vi "Untitled 1.vi"() -> ()   [LabVIEW 2016]
uses:
  Control 1.ctl
panel:
  out "Gauge":i32(knob) scale=0.0..100.0
  out "Numeric 2":dbl
  out "Numeric":T1
  in  "Slide":dbl(slide) scale=0.0..10.0
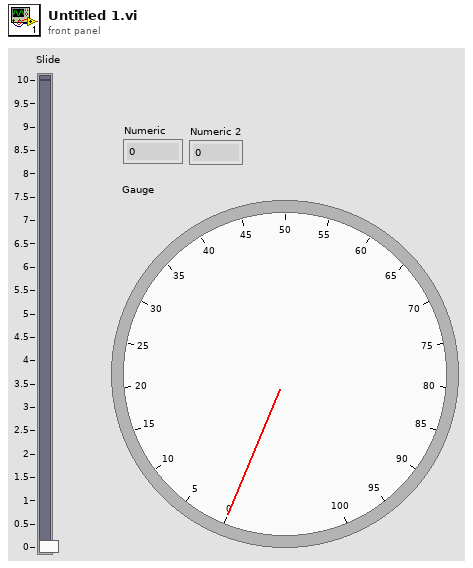
[diagram p1: front panel]
types:
  T1 = typedef "Control 1.ctl" = dbl
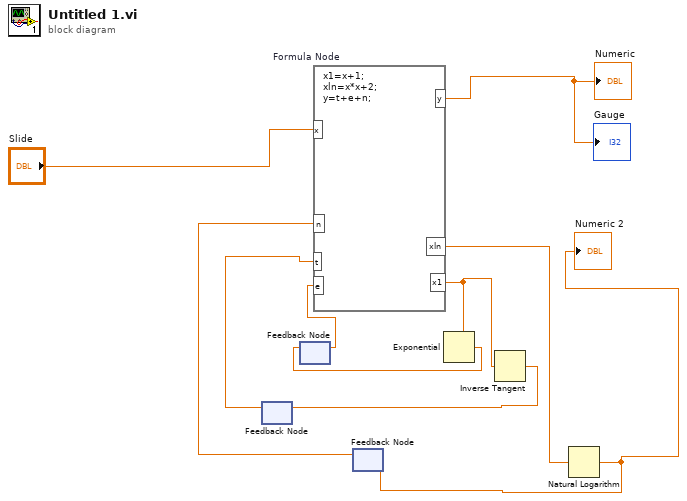
[diagram p0: block diagram]
diagram:
  n1 = feedback #1() -> (w3:dbl)  [unwired: 1 in]
  n2 = feedback #2() -> (w5:dbl)  [unwired: 1 in]
  n3 = feedback #3() -> (w2:dbl)  [unwired: 1 in]
  n4 = formula code="x1=x+1;\nxln=x*x+2;\ny=t+e+n;"("x"="Slide", "t"=w3, "e"=w5, "n"=w2) -> ("y"=→"Numeric" →"Gauge":dbl, "x1"=w7:dbl, "xln"=w8:dbl)
  n5 = Exponential(1:w7) -> (0:w6:dbl)
  n6 = feedback-in #2(w6) -> ()
  n7 = Inverse Tangent(1:w7) -> (0:w4:dbl)
  n8 = feedback-in #1(w4) -> ()
  n9 = Natural Logarithm(1:w8) -> (0:w1:dbl)
  "Numeric 2" <- w1
  n10 = feedback-in #3(w1) -> ()
